vi "MCP Close.vi"(8 "error in (no error)":errorcluster) -> (0 "error out":errorcluster)   [LabVIEW 2020]
uses:
  MCP2221A LabVIEW library/Microchip MCP2221A_64bit/VIs/Private/mcp2221_dll_um_x64.dll
panel:
  out "noOfDevs out":u32=1
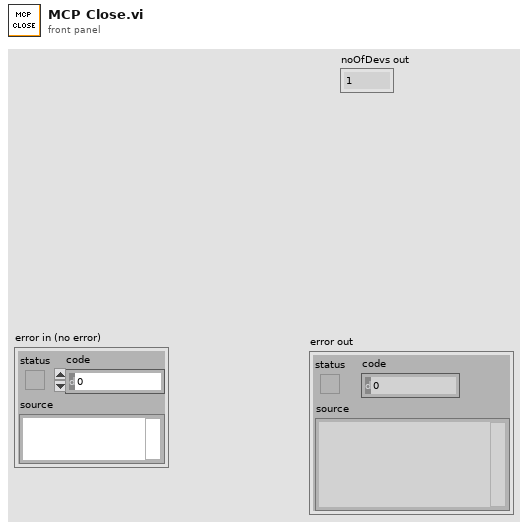
[diagram p1: front panel]
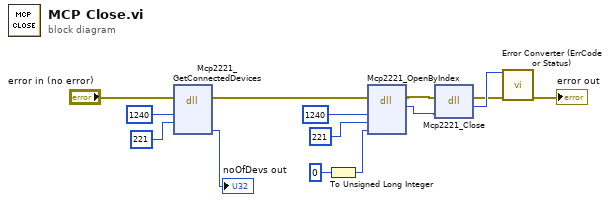
[diagram p0: block diagram]
diagram:
  n1 = dll-call lib="C:/Users/tuguialexand/Desktop/Licenta/MCP2221A LabVIEW library/Microchip MCP2221A_64bit/VIs/Private/mcp2221_dll_um_x64.dll" fn="Mcp2221_GetConnectedDevices"(error in="error in (no error)", "vid"=u32 1240, "pid"=u32 221) -> (error out=w5:errorcluster, "noOfDevs"=→"noOfDevs out":u32)  [unwired: 6 in, 1 out]
  n2 = To Unsigned Long Integer(number=0 ("index")) -> (unsigned 32bit integer=w8:u32)
  n3 = dll-call lib="C:/Users/tuguialexand/Desktop/Licenta/MCP2221A LabVIEW library/Microchip MCP2221A_64bit/VIs/Private/mcp2221_dll_um_x64.dll" fn="Mcp2221_OpenByIndex"(error in=w5, "VID"=u32 1240, "PID"=u32 221, "index"=w8) -> (error out=w1:errorcluster, "return type"=w2:u64)  [unwired: 5 in, 1 out]
  n4 = dll-call lib="C:/Users/tuguialexand/Desktop/Licenta/MCP2221A LabVIEW library/Microchip MCP2221A_64bit/VIs/Private/mcp2221_dll_um_x64.dll" fn="Mcp2221_Close"(error in=w1, "handle"=w2) -> (error out=w3:errorcluster, "return type"=w4:i32)  [unwired: 3 in, 1 out]
  n5 = call "Error Converter (ErrCode or Status).vi"("error code"=w4, "error in (no error)"=w3) -> ("error out"=→"error out":errorcluster)  [unwired: 13 in]
